vi "dfd_FXP PtByPt Direct IIR II.vi"(0 "x":T7={"value"=0, "wl"=0, "iwl"=0, "Signed"=TRUE} {"value" format="%.0x"}, 1 "quantizers":T5[](array[typedef]) {"source" items=["Coef a/k"=0, "Coef b/v"=7, "Input"=1, "Output"=2, "Multiplicand"=3, "Product"=4, "Sum"=5, "Delay"=6, "Gain"=8]}, 5 "coef b[0..M]":T4, 7 "coef a[1..N]":T4, 9 "state tmp in":i64[](array[numeric]), 11 "filtering statistics in":T3(array[cluster]) {"statistics information"."min value" format="%.2f"; "statistics information"."max value" format="%.2f"; "Quantizer Source" items=["Coefficients a/k"=0, "Coefficients b/v"=7, "Input"=1, "Output"=2, "Multiplicand"=3, "Product"=4, "Sum"=5, "Delay"=6]}, 12 "state in":i64[](array[numeric])) -> (4 "filtered x":T7={"value"=0, "wl"=0, "iwl"=0, "Signed"=TRUE} {"value" format="%.0x"}, 10 "state tmp out":i64[](array[numeric]), 14 "state out":i64[](array[numeric]), 15 "filtering statistics out":T3(array[cluster]) {"statistics information"."min value" format="%.2f"; "statistics information"."max value" format="%.2f"; "Quantizer Source" items=["Coefficients a/k"=0, "Coefficients b/v"=7, "Input"=1, "Output"=2, "Multiplicand"=3, "Product"=4, "Sum"=5, "Delay"=6]})   [LabVIEW 2017, in "NI_DigFilter_FXP.lvlib"]
uses:
  <vilib>/addons/Digital Filter Design/NI_DigFilter_FXP.lvlib
  <vilib>/addons/Digital Filter Design/_Objects.llb/dfd_DFXP Data Type (scaler).ctl
  <vilib>/addons/Digital Filter Design/_Objects.llb/dfd_DFXP Operation Parameter.ctl
  <vilib>/addons/Digital Filter Design/_Objects.llb/dfd_Internal Quantization Srcs.ctl
  <vilib>/addons/Digital Filter Design/_Objects.llb/dfd_DFXP Data Type (vector).ctl
  <vilib>/addons/Digital Filter Design/_Objects.llb/DFD Quantization Sources.ctl
  <vilib>/addons/Digital Filter Design/_Objects.llb/DFD FXP Statistics Data.ctl
  <vilib>/addons/Digital Filter Design/NI_DigFilterLicensed.lvlib
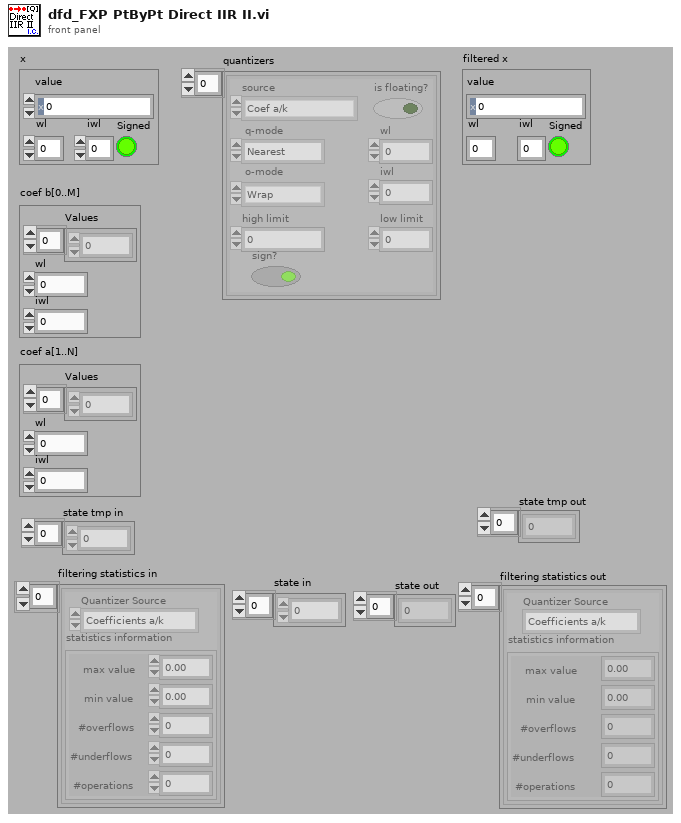
[diagram p1: front panel]
types:
  T1 = typedef "NI_DigFilterLicensed.lvlib/DFD Quantization Sources.ctl" = u16
  T2 = typedef "NI_DigFilterLicensed.lvlib/DFD FXP Statistics Data.ctl" = cluster{"max value":ext, "min value":ext, "#overflows":i32, "#underflows":i32, "#operations":i32}
  T3 = cluster{"Quantizer Source":T1, "statistics information":T2}[]
  T4 = typedef "dfd_DFXP Data Type (vector).ctl" = cluster{"Values":i64[], "wl":i16, "iwl":i16}
  T5 = typedef "dfd_DFXP Operation Parameter.ctl" = cluster{"source":T6, "is floating?":bool, "o-mode":enum16{"Saturation", "Wrap"}, "q-mode":enum16{"Nearest", "Truncation"}, "wl":i16, "high limit":i64, "low limit":i64, "iwl":i16, "sign?":bool}
  T6 = typedef "NI_DigFilterLicensed.lvlib/dfd_Internal Quantization Srcs.ctl" = u16
  T7 = typedef "dfd_DFXP Data Type (scaler).ctl" = cluster{"value":i64, "wl":i16, "iwl":i16, "Signed":bool}
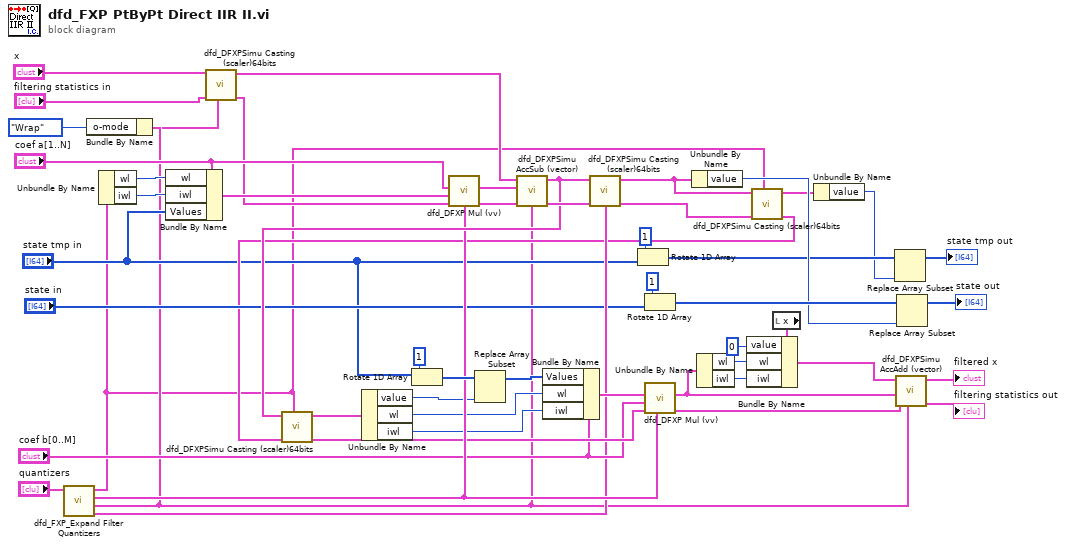
[diagram p0: block diagram]
diagram:
  n1 = call <vilib>:"dfd_FXP_Expand Filter Quantizers.vi"("FXPOPs"="quantizers") -> ("Delay"=w29:T5, "Sum"=w3:T5, "Product"=w41:T5, "Multiplicand"=w1:T5)  [unwired: 7 out]
  n2 = Bundle By Name(cluster=w3, "o-mode"=enum16{"Saturation", "Wrap"}."Wrap" ("overflow mode")) -> (w2:T5)
  n3 = Unbundle By Name(w1) -> ("wl"=w16:i16, "iwl"=w15:i16)
  n4 = Bundle By Name(cluster="coef a[1..N]", "wl"=w16, "iwl"=w15, "Values"="state tmp in") -> (w18:T4)
  n5 = call <vilib>:"dfd_DFXPSimu Casting (scaler)64bits.vi"("op params"=w2, "filtering statistics in"="filtering statistics in", "Value in"="x") -> ("filtering statistics out"=w7:T3, "Value out"=w8:T7)  [unwired: 1 in, 6 out]
  n6 = Rotate 1D Array(1:"state tmp in", 2:1 ("n")) -> (0:w42:i64[])
  n7 = call <vilib>:"dfd_DFXP Mul (vv).vi"("op params"=w41, "filtering statistics in"=w7, "Value in 2"=w18, "Value in"="coef a[1..N]") -> ("filtering statistics out"=w47:T3, "Value out"=w46:T4)  [unwired: 6 out]
  n8 = call <vilib>:"dfd_DFXPSimu AccSub (vector).vi"("op params"=w3, "filtering statistics in"=w47, "addends"=w46, "acc in"=w8) -> ("filtering statistics out"=w51:T3, "acc out"=w44:T7)  [unwired: 1 in, 5 out]
  n9 = call <vilib>:"dfd_DFXPSimu Casting (scaler)64bits.vi"("op params"=w29, "filtering statistics in"=w51, "Value in"=w44) -> ("filtering statistics out"=w20:T3, "Value out"=w21:T7)  [unwired: 1 in, 6 out]
  n10 = Rotate 1D Array(1:"state tmp in", 2:1 ("n")) -> (0:w13:i64[])
  n11 = Rotate 1D Array(1:"state in", 2:1 ("n")) -> (0:w45:i64[])
  n12 = Unbundle By Name(w21) -> ("value"=w30:i64)
  n13 = call <vilib>:"dfd_DFXPSimu Casting (scaler)64bits.vi"("op params"=w1, "filtering statistics in"=w20, "Value in"=w21) -> ("filtering statistics out"=w19:T3, "Value out"=w12:T7)  [unwired: 1 in, 6 out]
  n14 = call <vilib>:"dfd_DFXPSimu Casting (scaler)64bits.vi"("op params"=w1, "filtering statistics in"=w19, "Value in"=w44) -> ("filtering statistics out"=w40:T3, "Value out"=w37:T7)  [unwired: 1 in, 6 out]
  n15 = Unbundle By Name(w37) -> ("value"=w35:i64, "wl"=w32:i16, "iwl"=w31:i16)
  n16 = Replace Array Subset(array=w42, new element=w35) -> (w36:i64[])  [unwired: 1 in]
  n17 = Bundle By Name(cluster="coef b[0..M]", "Values"=w36, "wl"=w32, "iwl"=w31) -> (w34:T4)
  n18 = call <vilib>:"dfd_DFXP Mul (vv).vi"("op params"=w41, "filtering statistics in"=w40, "Value in 2"="coef b[0..M]", "Value in"=w34) -> ("filtering statistics out"=w49:T3, "Value out"=w28:T4)  [unwired: 6 out]
  n19 = Unbundle By Name(w28) -> ("wl"=w26:i16, "iwl"=w25:i16)
  n20 = local read "x"() -> (w27:T7)
  n21 = Bundle By Name(cluster=w27, "value"=i64 0, "wl"=w26, "iwl"=w25) -> (w23:T7)
  n22 = Unbundle By Name(w12) -> ("value"=w11:i64)
  n23 = Replace Array Subset(array=w13, new element=w11) -> (→"state tmp out":i64[])  [unwired: 1 in]
  n24 = call <vilib>:"dfd_DFXPSimu AccAdd (vector).vi"("op params"=w3, "filtering statistics in"=w49, "addends"=w28, "acc in"=w23) -> ("filtering statistics out"=→"filtering statistics out":T3, "acc out"=→"filtered x":T7)  [unwired: 1 in, 5 out]
  n25 = Replace Array Subset(array=w45, new element=w30) -> (→"state out":i64[])  [unwired: 1 in]
